vi "VISJS Viewer.vi"(4 "Extra Scripts":string, 5 "FileDependency In":map{path, T1}(c390), 6 "Options":string, 7 "OpenWebBrowser(False)":bool, 8 "error in":errorcluster, 9 "Embedd VISJS Librarya in HTMl File(False)":bool, 10 "HTMLFilePath":path, 11 "LibraryDependency":map{path, T3}(c390)) -> (0 "error out":errorcluster, 3 "HTMLFileContent":string)   [LabVIEW 2020, in "VISJS Viewer.lvlib"] (continued)
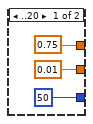
[diagram p2: hidden frame]
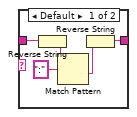
[diagram p7: hidden frame]
d=r[2];e<s&&(e=s,C=n,I=a,i=d)}}return[C,e,I,i]}},{key:\"_getEnergy\",value:function(g){var t=lh(this.E_sums[g],2),A=t[0],e=t[1];return[Math.sqrt(Math.pow(A,2)+Math.pow(e,2)),A,e]}},{key:\"_moveNode\",value:function(g,t,A){for(var e=this.body.nodeIndices,C=this.body.nodes,I=0,i=0,o=0,n=C[g].x,r=C[g].y,s=this.K_matrix[g],a=this.L_matrix[g],d=0;d<e.length;d++){var h=e[d];if(h!==g){var l=C[h].x,c=C[h].y,u=s[h],p=a[h],f=1/Math.pow(Math.pow(n-l,2)+Math.pow(r-c,2),1.5);I+=u*(1-p*Math.pow(r-c,2)*f),i+=u*(p*(n-l)*(r-c)*f),o+=u*(1-p*Math.pow(n-l,2)*f)}}var v=(t/I+A/i)/(i/I-o/i),y=-(i*v+t)/I;C[g].x+=y,C[g].y+=v,this._updateE_matrix(g)}},{key:\"_createL_matrix\",value:function(g){var t=this.body.nodeIndices,A=this.springLength;this.L_matrix=[];for(var e=0;e<t.length;e++){this.L_matrix[t[e]]={};for(var C=0;C<t.length;C++)this.L_matrix[t[e]][t[C]]=A*g[t[e]][t[C]]}}},{key:\"_createK_matrix\",value:function(g){var t=this.body.nodeIndices,A=this.springConstant;this.K_matrix=[];for(var e=0;e<t.length;e++){this.K_matrix[t[e]]={};for(var C=0;C<t.length;C++)this.K_matrix[t[e]][t[C]]=A*Math.pow(g[t[e]][t[C]],-2)}}},{key:\"_createE_matrix\",value:function(){var g=this.body.nodeIndices,t=this.body.nodes;this.E_matrix={},this.E_sums={};for(var A=0;A<g.length;A++)this.E_matrix[g[A]]=[];for(var e=0;e<g.length;e++){for(var C=g[e],I=t[C].x,i=t[C].y,o=0,n=0,r=e;r<g.length;r++){var s=g[r];if(s!==C){var a=t[s].x,d=t[s].y,h=1/Math.sqrt(Math.pow(I-a,2)+Math.pow(i-d,2));this.E_matrix[C][r]=[this.K_matrix[C][s]*(I-a-this.L_matrix[C][s]*(I-a)*h),this.K_matrix[C][s]*(i-d-this.L_matrix[C][s]*(i-d)*h)],this.E_matrix[s][e]=this.E_matrix[C][r],o+=this.E_matrix[C][r][0],n+=this.E_matrix[C][r][1]}}this.E_sums[C]=[o,n]}}},{key:\"_updateE_matrix\",value:function(g){for(var t=this.body.nodeIndices,A=this.body.nodes,e=this.E_matrix[g],C=this.K_matrix[g],I=this.L_matrix[g],i=A[g].x,o=A[g].y,n=0,r=0,s=0;s<t.length;s++){var a=t[s];if(a!==g){var d=e[s],h=d[0],l=d[1],c=A[a].x,u=A[a].y,p=1/Math.sqrt(Math.pow(i-c,2)+Math.pow(o-u,2)),f=C[a]*(i-c-I[a]*(i-c)*p),v=C[a]*(o-u-I[a]*(o-u)*p);e[s]=[f,v],n+=f,r+=v;var y=this.E_sums[a];y[0]+=f-h,y[1]+=v-l}}this.E_sums[g]=[n,r]}}]),g}();function gB(g,t,A){var e,C,I,i,o=this;if(!(this instanceof gB))throw new SyntaxError(\"Constructor must be called with the new operator\");this.options={},this.defaultOptions={locale:\"en\",locales:ny,clickToUse:!1},fe(this.options,this.defaultOptions),this.body={container:g,nodes:{},nodeIndices:[],edges:{},edgeIndices:[],emitter:{on:je(e=this.on).call(e,this),off:je(C=this.off).call(C,this),emit:je(I=this.emit).call(I,this),once:je(i=this.once).call(i,this)},eventListeners:{onTap:function(){},onTouch:function(){},onDoubleTap:function(){},onHold:function(){},onDragStart:function(){},onDrag:function(){},onDragEnd:function(){},onMouseWheel:function(){},onPinch:function(){},onMouseMove:function(){},onRelease:function(){},onContext:function(){}},data:{nodes:null,edges:null},functions:{createNode:function(){},createEdge:function(){},getPointer:function(){}},modules:{},view:{scale:1,translation:{x:0,y:0}},selectionBox:{show:!1,position:{start:{x:0,y:0},end:{x:0,y:0}}}},this.bindEventListeners(),this.images=new sy((function(){return o.body.emitter.emit(\"_requestRedraw\")})),this.groups=new Gm,this.canvas=new CP(this.body),this.selectionHandler=new yM(this.body,this.canvas),this.interactionHandler=new sP(this.body,this.canvas,this.selectionHandler),this.view=new IP(this.body,this.canvas),this.renderer=new gP(this.body,this.canvas),this.physics=new HR(this.body),this.layoutEngine=new ZM(this.body),this.clustering=new $R(this.body),this.manipulation=new jM(this.body,this.canvas,this.selectionHandler,this.interactionHandler),this.nodesHandler=new YN(this.body,this.images,this.groups,this.layoutEngine),this.edgesHandler=new FR(this.body,this.images,this.groups),this.body.modules.kamadaKawai=new $M(this.body,150,.05),this.body.modules.clustering=this.clustering,this.canvas._create(),this.setOptions(A),this.setData(t)}He(gB.prototype),gB.prototype.setOptions=function(g){var t=this;if(null===g&&(g=void 0),void 0!==g){!0===Dv.validate(g,KM)&&console.error(\"%cErrors have been found in the supplied options object.\",Tv);if(Xf([\"locale\",\"locales\",\"clickToUse\"],this.options,g),void 0!==g.locale&&(g.locale=function(g,t){try{var A=lh(t.split(/[-_ /]/,2),2),e=A[0],C=A[1],I=null!=e?e.toLowerCase():null,i=null!=C?C.toUpperCase():null;if(I&&i){var o,n=I+\"-\"+i;if(Object.prototype.hasOwnProperty.call(g,n))return n;console.warn(bh(o=\"Unknown variant \".concat(i,\" of language \")).call(o,I,\".\"))}if(I){var r=I;if(Object.prototype.hasOwnProperty.call(g,r))return r;console.warn(\"Unknown language \".concat(I))}return console.warn(\"Unknown locale \".concat(t,\", falling back to English.\")),\"en\"}catch(g){return console.error(g),console.warn(\"Unexpected error while normalizing locale \".concat(t,\", falling back to English.\")),\"en\"}}(g.locales||this.options.locales,g.locale)),g=this.layoutEngine.setOptions(g.layout,g),this.canvas.setOptions(g),this.groups.setOptions(g.groups),this.nodesHandler.setOptions(g.nodes),this.edgesHandler.setOptions(g.edges),this.physics.setOptions(g.physics),this.manipulation.setOptions(g.manipulation,g,this.options),this.interactionHandler.setOptions(g.interaction),this.renderer.setOptions(g.interaction),this.selectionHandler.setOptions(g.interaction),void 0!==g.groups&&this.body.emitter.emit(\"refreshNodes\"),\"configure\"in g&&(this.configurator||(this.configurator=new xv(this,this.body.container,HM,this.canvas.pixelRatio,XM)),this.configurator.setOptions(g.configure)),this.configurator&&!0===this.configurator.options.enabled){var A={nodes:{},edges:{},layout:{},interaction:{},manipulation:{},physics:{},global:{}};qf(A.nodes,this.nodesHandler.options),qf(A.edges,this.edgesHandler.options),qf(A.layout,this.layoutEngine.options),qf(A.interaction,this.selectionHandler.options),qf(A.interaction,this.renderer.options),qf(A.interaction,this.interactionHandler.options),qf(A.manipulation,this.manipulation.options),qf(A.physics,this.physics.options),qf(A.global,this.canvas.options),qf(A.global,this.options),this.configurator.setModuleOptions(A)}void 0!==g.clickToUse?!0===g.clickToUse?void 0===this.activator&&(this.activator=new kv(this.canvas.frame),this.activator.on(\"change\",(function(){t.body.emitter.emit(\"activate\")}))):(void 0!==this.activator&&(this.activator.destroy(),delete this.activator),this.body.emitter.emit(\"activate\")):this.body.emitter.emit(\"activate\"),this.canvas.setSize(),this.body.emitter.emit(\"startSimulation\")}},gB.prototype._updateVisibleIndices=function(){var g=this.body.nodes,t=this.body.edges;for(var A in this.body.nodeIndices=[],this.body.edgeIndices=[],g)Object.prototype.hasOwnProperty.call(g,A)&&(this.clustering._isClusteredNode(A)||!1!==g[A].options.hidden||this.body.nodeIndices.push(g[A].id));for(var e in t)if(Object.prototype.hasOwnProperty.call(t,e)){var C=t[e],I=g[C.fromId],i=g[C.toId],o=void 0!==I&&void 0!==i;!this.clustering._isClusteredEdge(e)&&!1===C.options.hidden&&o&&!1===I.options.hidden&&!1===i.options.hidden&&this.body.edgeIndices.push(C.id)}},gB.prototype.bindEventListeners=function(){var g=this;this.body.emitter.on(\"_dataChanged\",(function(){g.edgesHandler._updateState(),g.body.emitter.emit(\"_dataUpdated\")})),this.body.emitter.on(\"_dataUpdated\",(function(){g.clustering._updateState(),g._updateVisibleIndices(),g._updateValueRange(g.body.nodes),g._updateValueRange(g.body.edges),g.body.emitter.emit(\"startSimulation\"),g.body.emitter.emit(\"_requestRedraw\")}))},gB.prototype.setData=function(g){if(this.body.emitter.emit(\"resetPhysics\"),this.body.emitter.emit(\"_resetData\"),this.selectionHandler.unselectAll(),g&&g.dot&&(g.nodes||g.edges))throw new SyntaxError('Data must contain either parameter \"dot\" or  parameter pair \"nodes\" and \"edges\", but not both.');if(this.setOptions(g&&g.options),g&&g.dot){console.warn(\"The dot property has been deprecated. Please use the static convertDot method to convert DOT into vis.network format and use the normal data format with nodes and edges. This converter is used like this: var data = vis.network.convertDot(dotString);\");var t=Cy(g.dot);this.setData(t)}else if(g&&g.gephi){console.warn(\"The gephi property has been deprecated. Please use the static convertGephi method to convert gephi into vis.network format and use the normal data format with nodes and edges. This converter is used like this: var data = vis.network.convertGephi(gephiJson);\");var A=iy(g.gephi);this.setData(A)}else this.nodesHandler.setData(g&&g.nodes,!0),this.edgesHandler.setData(g&&g.edges,!0),this.body.emitter.emit(\"_dataChanged\"),this.body.emitter.emit(\"_dataLoaded\"),this.body.emitter.emit(\"initPhysics\")},gB.prototype.destroy=function(){for(var g in this.body.emitter.emit(\"destroy\"),this.body.emitter.off(),this.off(),delete this.groups,delete this.canvas,delete this.selectionHandler,delete this.interactionHandler,delete this.view,delete this.renderer,delete this.physics,delete this.layoutEngine,delete this.clustering,delete this.manipulation,delete this.nodesHandler,delete this.edgesHandler,delete this.configurator,delete this.images,this.body.nodes)Object.prototype.hasOwnProperty.call(this.body.nodes,g)&&delete this.body.nodes[g];for(var t in this.body.edges)Object.prototype.hasOwnProperty.call(this.body.edges,t)&&delete this.body.edges[t];Qf(this.body.container)},gB.prototype._updateValueRange=function(g){var t,A=void 0,e=void 0,C=0;for(t in g)if(Object.prototype.hasOwnProperty.call(g,t)){var I=g[t].getValue();void 0!==I&&(A=void 0===A?I:Math.min(I,A),e=void 0===e?I:Math.max(I,e),C+=I)}if(void 0!==A&&void 0!==e)for(t in g)Object.prototype.hasOwnProperty.call(g,t)&&g[t].setValueRange(A,e,C)},gB.prototype.isActive=function(){return!this.activator||this.activator.active},gB.prototype.setSize=function(){return this.canvas.setSize.apply(this.canvas,arguments)},gB.prototype.canvasToDOM=function(){return this.canvas.canvasToDOM.apply(this.canvas,arguments)},gB.prototype.DOMtoCanvas=function(){return this.canvas.DOMtoCanvas.apply(this.canvas,arguments)},gB.prototype.findNode=function(){return this.clustering.findNode.apply(this.clustering,arguments)},gB.prototype.isCluster=function(){return this.clustering.isCluster.apply(this.clustering,arguments)},gB.prototype.openCluster=function(){return this.clustering.openCluster.apply(this.clustering,arguments)},gB.prototype.cluster=function(){return this.clustering.cluster.apply(this.clustering,arguments)},gB.prototype.getNodesInCluster=function(){return this.clustering.getNodesInCluster.apply(this.clustering,arguments)},gB.prototype.clusterByConnection=function(){return this.clustering.clusterByConnection.apply(this.clustering,arguments)},gB.prototype.clusterByHubsize=function(){return this.clustering.clusterByHubsize.apply(this.clustering,arguments)},gB.prototype.updateClusteredNode=function(){return this.clustering.updateClusteredNode.apply(this.clustering,arguments)},gB.prototype.getClusteredEdges=function(){return this.clustering.getClusteredEdges.apply(this.clustering,arguments)},gB.prototype.getBaseEdge=function(){return this.clustering.getBaseEdge.apply(this.clustering,arguments)},gB.prototype.getBaseEdges=function(){return this.clustering.getBaseEdges.apply(this.clustering,arguments)},gB.prototype.updateEdge=function(){return this.clustering.updateEdge.apply(this.clustering,arguments)},gB.prototype.clusterOutliers=function(){return this.clustering.clusterOutliers.apply(this.clustering,arguments)},gB.prototype.getSeed=function(){return this.layoutEngine.getSeed.apply(this.layoutEngine,arguments)},gB.prototype.enableEditMode=function(){return this.manipulation.enableEditMode.apply(this.manipulation,arguments)},gB.prototype.disableEditMode=function(){return this.manipulation.disableEditMode.apply(this.manipulation,arguments)},gB.prototype.addNodeMode=function(){return this.manipulation.addNodeMode.apply(this.manipulation,arguments)},gB.prototype.editNode=function(){return this.manipulation.editNode.apply(this.manipulation,arguments)},gB.prototype.editNodeMode=function(){return console.warn(\"Deprecated: Please use editNode instead of editNodeMode.\"),this.manipulation.editNode.apply(this.manipulation,arguments)},gB.prototype.addEdgeMode=function(){return this.manipulation.addEdgeMode.apply(this.manipulation,arguments)},gB.prototype.editEdgeMode=function(){return this.manipulation.editEdgeMode.apply(this.manipulation,arguments)},gB.prototype.deleteSelected=function(){return this.manipulation.deleteSelected.apply(this.manipulation,arguments)},gB.prototype.getPositions=function(){return this.nodesHandler.getPositions.apply(this.nodesHandler,arguments)},gB.prototype.getPosition=function(){return this.nodesHandler.getPosition.apply(this.nodesHandler,arguments)},gB.prototype.storePositions=function(){return this.nodesHandler.storePositions.apply(this.nodesHandler,arguments)},gB.prototype.moveNode=function(){return this.nodesHandler.moveNode.apply(this.nodesHandler,arguments)},gB.prototype.getBoundingBox=function(){return this.nodesHandler.getBoundingBox.apply(this.nodesHandler,arguments)},gB.prototype.getConnectedNodes=function(g){return void 0!==this.body.nodes[g]?this.nodesHandler.getConnectedNodes.apply(this.nodesHandler,arguments):this.edgesHandler.getConnectedNodes.apply(this.edgesHandler,arguments)},gB.prototype.getConnectedEdges=function(){return this.nodesHandler.getConnectedEdges.apply(this.nodesHandler,arguments)},gB.prototype.startSimulation=function(){return this.physics.startSimulation.apply(this.physics,arguments)},gB.prototype.stopSimulation=function(){return this.physics.stopSimulation.apply(this.physics,arguments)},gB.prototype.stabilize=function(){return this.physics.stabilize.apply(this.physics,arguments)},gB.prototype.getSelection=function(){return this.selectionHandler.getSelection.apply(this.selectionHandler,arguments)},gB.prototype.setSelection=function(){return this.selectionHandler.setSelection.apply(this.selectionHandler,arguments)},gB.prototype.getSelectedNodes=function(){return this.selectionHandler.getSelectedNodeIds.apply(this.selectionHandler,arguments)},gB.prototype.getSelectedEdges=function(){return this.selectionHandler.getSelectedEdgeIds.apply(this.selectionHandler,arguments)},gB.prototype.getNodeAt=function(){var g=this.selectionHandler.getNodeAt.apply(this.selectionHandler,arguments);return void 0!==g&&void 0!==g.id?g.id:g},gB.prototype.getEdgeAt=function(){var g=this.selectionHandler.getEdgeAt.apply(this.selectionHandler,arguments);return void 0!==g&&void 0!==g.id?g.id:g},gB.prototype.selectNodes=function(){return this.selectionHandler.selectNodes.apply(this.selectionHandler,arguments)},gB.prototype.selectEdges=function(){return this.selectionHandler.selectEdges.apply(this.selectionHandler,arguments)},gB.prototype.unselectAll=function(){this.selectionHandler.unselectAll.apply(this.selectionHandler,arguments),this.selectionHandler.commitWithoutEmitting.apply(this.selectionHandler),this.redraw()},gB.prototype.redraw=function(){return this.renderer.redraw.apply(this.renderer,arguments)},gB.prototype.getScale=function(){return this.view.getScale.apply(this.view,arguments)},gB.prototype.getViewPosition=function(){return this.view.getViewPosition.apply(this.view,arguments)},gB.prototype.fit=function(){return this.view.fit.apply(this.view,arguments)},gB.prototype.moveTo=function(){return this.view.moveTo.apply(this.view,arguments)},gB.prototype.focus=function(){return this.view.focus.apply(this.view,arguments)},gB.prototype.releaseNode=function(){return this.view.releaseNode.apply(this.view,arguments)},gB.prototype.getOptionsFromConfigurator=function(){var g={};return this.configurator&&(g=this.configurator.getOptions.apply(this.configurator)),g};var tB=Cy;g.DataSet=mD,g.DataView=bD,g.Network=gB,g.NetworkImages=sy,g.Queue=fD,g.data=xD,g.networkDOTParser=Iy,g.networkGephiParser=oy,g.networkOptions=JM,g.parseDOTNetwork=tB,g.parseGephiNetwork=iy}));\n//# sourceMappingURL=vis-network.min.js.map\n"  # https://visjs.github.io/vis-network/standalone/umd/vis-network.min.js 2024-08-26T06:20:20.413Z
  n1 = Array Size(array=w28) -> (size(s)=w29:i32)
  n2 = for {
    tunnel: "LibraryDependency" -> [w51] mode=indexing
    tunnel: "{from: \"%s\",to: \"%s\",arrows: \"to\",id: \"E%d\"}\n" -> [w49]
    tunnel: [w44] -> w25 mode=concatenating
    shift-right: [w42] -> _
    shift-left: 0 -> [w48]
    tunnel: "FileDependency In" -> [w47]
    tunnel: [w43] -> w4 mode=concatenating
    tunnel: [w46] -> _ mode=indexing
    i -> [w46]
    n3 = Unbundle By Name(w51) -> ("LibraryDependentInfo.ParentLibraries"=w41:path[], "Path"=w45:path, "LibraryDependentInfo.DependentLibrary"=w50:map{path, set{path}})  [unwired: 1 out]
    n4 = for {
      tunnel: w45 -> [w72]
      tunnel: w50 -> [w69] mode=indexing
      tunnel: w49 -> [w71]
      tunnel: [w70] -> w44 mode=indexing
      shift-right: [w55] -> w42
      shift-left: w48 -> [w66]
      tunnel: w47 -> [w65]
      tunnel: [w62] -> w43 mode=indexing
      tunnel: w41 -> [w57]
      n5 = Unbundle By Name(w69) -> ("Path"=w56:path, "Callers"=w64:set{path})
      n6 = for {
        tunnel: w65 -> [w98]
        tunnel: w64 -> [w97] mode=indexing
        shift-right: [w93] -> w60
        shift-left: map{string, set{string}} {} ("Size: 0") -> [w95]
        n7 = Look In Map(map=w98, key=w97) -> (value=w96:T1)  [unwired: 1 in, 1 out]
        n8 = Unbundle By Name(w96) -> ("FullQualifierName"=w90:string, "Path"=w92:path)
        n9 = call <vilib>:"Get File Extension.vi"("file"=w92) -> ("lowercase file extension"=w91:string)  [unwired: 6 in, 4 out]
        n10 = case shown="\"lvclass\"" w91 {
          tunnel: w90 -> [w103 w104]
          tunnel: [w99 w104] -> w89
          frame Default {
            n11 = Reverse String(1:w103) -> (0:w102:string)
            n12 = Match Pattern(string=w102, regular expression=":") -> (after substring=w100:string)  [unwired: 1 in, 3 out]
            n13 = Reverse String(1:w100) -> (0:w99:string)
          }
          frame "lvclass" {
          }
        }
        n14 = Strip Path(path=w92) -> (name=w94:string)  [unwired: 1 out]
        n15 = in-place {
          in-place-border: w94 -> [w107]
          n16 = in-place-map #1(w95, w89) -> (w108:set{string})  [unwired: 1 in, 1 out]
          n17 = Insert Into Set(10:w107, 11:w108) -> (3:w106:set{string})  [unwired: 1 out]
          n18 = in-place-map #1(w106, LVMapReplaceAction."Add or Modify Entry" ("action")) -> (w93:map{string, set{string}})  [unwired: 2 out]
        }
      }
      n19 = Search 1D Array(1D array=w57, element=w56) -> (index of element=w53:i32)  [unwired: 1 in]
      n20 = case shown="0, Default" w53 {
        tunnel: ["INHERITANCE " _] -> w52
        frame 0, Default {
        }
        frame -1 {
        }
      }
      n21 = Increment(x=w66) -> (x+1=w55:i32)
      n22 = for {
        tunnel: w60 -> [w80] mode=indexing
        tunnel: [w77] -> w59 mode=indexing
        n23 = Unbundle(w80) -> ("FullQualifierName"=w75:string, w79:set{string})
        n24 = for {
          tunnel: w79 -> [w88] mode=indexing
          tunnel: [w88] -> w78 mode=indexing if=w86
          tunnel: w75 -> [w87]
          n25 = Not Equal?(x=w87, y=w88) -> (x != y?=w86:bool)
        }
        n26 = call <vilib>:"Join Strings.vi"("Separator (,)"=", ", "Strings In"=w78) -> ("String"=w76:string)  [unwired: 1 in]
        n27 = case shown="Default" w75 {
          selector: w75 -> [_ w85]
          tunnel: w76 -> [w81 w83]
          tunnel: [w81 w82] -> w77
          frame "" {
          }
          frame Default {
            n28 = Format Into String(format string="%s  [%s]", w85, w83) -> (resulting string=w82:string)  [unwired: 2 in, 1 out]
          }
        }
      }
      n29 = call "VISJS Viewer_EscapePath.vi"("Path"=w72) -> ("File Path"=w68:string)  [unwired: 10 in]
      n30 = call "VISJS Viewer_EscapePath.vi"("Path"=w56) -> ("File Path"=w67:string)  [unwired: 10 in]
      n31 = call <vilib>:"Join Strings.vi"("Separator (,)"="<BR> ", "Strings In"=w59) -> ("String"=w54:string)  [unwired: 1 in]
      n32 = Format Into String(format string="E%d : \"%s%s\"\n", w55, w52, w54) -> (resulting string=w62:string)  [unwired: 2 in, 1 out]
      n33 = Format Into String(format string=w71, w68, w67, w55) -> (resulting string=w70:string)  [unwired: 2 in, 1 out]
    }
  }
  n34 = for {
    tunnel: "LibraryDependency" -> [w127] mode=indexing
    tunnel: "{id: \"%s\",size: 150,label:\"%s\",color: \"#%02X%02X%02x\",cid: \"%s\",shape: \"box\"}\n" -> [w126]
    tunnel: w29 -> [w124]
    tunnel: w28 -> [w122]
    tunnel: [w116] -> w27 mode=indexing
    i -> [w125]
    w110 = ":" ("search string")
    n35 = Unbundle By Name(w127) -> ("Path"=w121:path, "LibraryDependentInfo.FullQualifierName"=w111:string)
    n36 = Quotient & Remainder(x=w125, y=w124) -> (x-y*floor(x/y)=w123:i32)  [unwired: 1 out]
    n37 = Index Array(array=w122, index=w123) -> (element=w120:u32)
    n38 = call <vilib>:"Color to RGB.vi"("Color"=w120) -> ("R"=w119:u8, "G"=w118:u8, "B"=w117:u8)  [unwired: 1 out]
    n39 = Match Pattern(string=w111, regular expression=w110) -> (before substring=w109:string)  [unwired: 1 in, 3 out]
    n40 = Search and Replace String(replace all?=TRUE ("replace all? (F)"), input string=w111, search string=w110, replace string="\\n" ("replace string (\"\")")) -> (result string=w113:string)  [unwired: 4 in, 3 out]
    n41 = call "VISJS Viewer_EscapePath.vi"("Path"=w121) -> ("File Path"=w115:string)  [unwired: 10 in]
    n42 = Format Into String(format string=w126, w115, w113, w119, w118, w117, w109) -> (resulting string=w116:string)  [unwired: 2 in, 1 out]
  }
  n43 = Empty String/Path?(string/path="HTMLFilePath") -> (empty?=w36:bool)
  n44 = Compound Arithmetic op=AND(w36, "OpenWebBrowser(False)") -> (w35:bool)
  n45 = Collection Size(1:"LibraryDependency") -> (0:w11:i32)
  n46 = case shown="21.." w11 {
    tunnel: [0.75 0.75] -> w8
    tunnel: [0.01 0.01] -> w7
    tunnel: [50 125] -> w6
    frame ..20 {
    }
    frame 21.. {
    }
  }
  n47 = case shown="True" w35 {
    tunnel: "HTMLFilePath" -> [w134 _]
    tunnel: [w134 w135] -> w18
    frame False {
    }
    frame True {
      n48 = Temporary Directory() -> (w137:path)
      n49 = Build Path(base path=w137, name or relative path=path "VISJS_Viewer.html") -> (appended path=w135:path)
    }
  }
  n50 = Format Into String(format string=w9, w8, w7, w6) -> (resulting string=w10:string)  [unwired: 2 in, 1 out]
  n51 = call <vilib>:"Join Strings.vi"("Strings In"=w27) -> ("String"=w26:string)  [unwired: 2 in]
  n52 = Select(t=w39, s="Embedd VISJS Librarya in HTMl File(False)", f="<script src=\"https://visjs.github.io/vis-network/standalone/umd/vis-network.min.js\"></script>") -> (s? t:f=w32:string)
  n53 = Empty String/Path?(string/path="Options") -> (empty?=w15:bool)
  n54 = Select(t=w10, s=w15, f="Options") -> (s? t:f=w13:string)
  n55 = call <vilib>:"Join Strings.vi"("Strings In"=w25) -> ("String"=w24:string)  [unwired: 2 in]
  n56 = call <vilib>:"Join Strings.vi"("Strings In"=w4) -> ("String"=w3:string)  [unwired: 2 in]
  n57 = Build Array(w32, w13, w26, w24, "Extra Scripts", w3) -> (w31:string[])
  n58 = for {
    shift-right: [w140] -> w17
    shift-left: "\n<html lang=\"en\">\n  <head>\n    <title>Vis Network | Example Applications | Disassembler</title>\n    <style type=\"text/css\">\n      #mynetwork {\n        width: 100%;\n        height: 80vh; /* Adjust height so the information appears at the bottom */\n        border: 0px solid lightgray;\n      }\n      #edgeInfo {\n        padding: 10px;\n        background-color: #f9f9f9;\n        border-top: 1px solid #ddd;\n      }\n\n /* Context menu styles */\n    .context-menu {\n      position: absolute;\n      display: none;\n      background-color: white;\n      border: 1px solid #ccc;\n      z-index: 100;\n      padding: 10px;\n      box-shadow: 2px 2px 5px rgba(0,0,0,0.2);\n    }\n\n    .context-menu button {\n      display: block;\n      background: none;\n      border: none;\n      padding: 5px 10px;\n      text-align: left;\n      width: 100%;\n      cursor: pointer;\n    }\n\n    .context-menu button:hover {\n      background-color: #f1f1f1;\n    }\n\n    #selectionBox {\n      position: absolute;\n      border: 1px dashed #555;\n      background: rgba(0, 0, 255, 0.1);\n      display: none;\n    }\n    </style>\n    <<VISJS>>\n  </head>\n  <body>\n    <div id=\"mynetwork\"></div>\n    <div id=\"selectionBox\"></div>\n    <div id=\"contextMenu\" class=\"context-menu\">\n      <button id=\"togglePhysics\">Toggle Physics</button>\n    </div>\n    <div id=\"edgeInfo\">Click on a node or edge to view its dependency details.<BR>Right-click on a node to turn the physics on or off for that node.<BR>To select multiple nodes, hold Shift and drag with a left click.</div>\n    <script type=\"text/javascript\">\n\nconst options = {\n<<OPTIONS>>\n};\n\nvar nodes = new vis.DataSet([\n<<NODES>>\n]);\n\n\nvar edges = new vis.DataSet([\n<<EDGES>>\n]);\n\nconst edgeInfoMap = {\n <<EDGEDEPENDECY>>\n};\n\n\n      var container = document.getElementById(\"mynetwork\");\n      var data = { nodes: nodes, edges: edges };\n      var gph = new vis.Network(container, data, options);\n      var contextMenu = document.getElementById('contextMenu');\n      var selectedNodeId = null;\n      var selectionBox = document.getElementById('selectionBox');\n      var startX, startY, isSelecting = false;\n\n      // Show context menu on right-click\n      gph.on(\"oncontext\", function (params) {\n        params.event.preventDefault();\n        var nodeId = gph.getNodeAt(params.pointer.DOM);\n\n        if (nodeId !== undefined) {\n          selectedNodeId = nodeId;\n          contextMenu.style.left = params.event.pageX + \"px\";\n          contextMenu.style.top = params.event.pageY + \"px\";\n          contextMenu.style.display = \"block\";\n        }\n      });\n\n      // Hide context menu when clicking anywhere\n      document.addEventListener(\"click\", function () {\n        contextMenu.style.display = \"none\";\n      });\n\n    document.getElementById('togglePhysics').addEventListener('click', function () {\n        if (selectedNodeId !== null) {\n        var node = nodes.get(selectedNodeId);\n        \n        // Toggle the physics state\n        if (node.physics === undefined || node.physics === null) node.physics = true;\n        node.physics = !node.physics;\n\n        // Update the node with the new fixed state\n                nodes.update(node);\n\n        selectedNodeId = null;\n        contextMenu.style.display = \"none\";\n        }\n    });\n\n    // Capture mousedown to start selection\n    container.addEventListener('mousedown', function(event) {\n    startX = event.clientX;\n    startY = event.clientY;\n    selectionBox.style.left = startX + 'px';\n    selectionBox.style.top = startY + 'px';\n    selectionBox.style.width = '0px';\n    selectionBox.style.height = '0px';\n    selectionBox.style.display = 'block';\n    isSelecting = true;\n  });\n\n  // Capture mousemove to draw the selection box\n  container.addEventListener('mousemove', function(event) {\n    if (isSelecting) {\n      var currentX = event.clientX;\n      var currentY = event.clientY;\n      selectionBox.style.left = Math.min(startX, currentX) + 'px';\n      selectionBox.style.top = Math.min(startY, currentY) + 'px';\n      selectionBox.style.width = Math.abs(currentX - startX) + 'px';\n      selectionBox.style.height = Math.abs(currentY - startY) + 'px';\n    }\n  });\n\n  // Capture mouseup to end selection and select nodes\n  container.addEventListener('mouseup', function(event) {\n    if (isSelecting) {\n      var endX = event.clientX;\n      var endY = event.clientY;\n\n      var selectionRect = {\n        left: Math.min(startX, endX),\n        right: Math.max(startX, endX),\n        top: Math.min(startY, endY),\n        bottom: Math.max(startY, endY)\n      };\n\n      var selectedNodes = [];\n      nodes.forEach(function(node) {\n        var nodePosition = gph.getPositions([node.id])[node.id];\n        var canvasPosition = gph.canvasToDOM(nodePosition);\n\n        // Check if node is inside the selection box\n        if (canvasPosition.x >= selectionRect.left && canvasPosition.x <= selectionRect.right &&\n            canvasPosition.y >= selectionRect.top && canvasPosition.y <= selectionRect.bottom) {\n          selectedNodes.push(node.id);\n        }\n      });\n\n      // Highlight selected nodes\n      gph.selectNodes(selectedNodes);\n      selectionBox.style.display = 'none';\n      isSelecting = false;\n    }\n  });\n\n  // Optional: Reset selection box on mouse leave\n  container.addEventListener('mouseleave', function() {\n    selectionBox.style.display = 'none';\n    isSelecting = false;\n  });\n/*\ngph.fit({\n animation: false, // Smooth transition\n minZoomLevel: .1, // Prevent zooming out too far\n maxZoomLevel: 10  // Allow zooming in more\n});\n*/\n   gph.on(\"click\", function (params) {\n  const edgeInfoElement = document.getElementById(\"edgeInfo\");\n  \n  // Check if a node is clicked\n  const nodeId = this.getNodeAt(params.pointer.DOM);\n  if (nodeId) {\n    // Get all edges where the nodeId is the \"from\" node\n    const connectedEdges = edges.get({\n      filter: (edge) => edge.from === nodeId,\n    });\n\nif (connectedEdges.length > 0) {\n  let allEdgeInfo = \"\";\n  connectedEdges.forEach((edge, index) => {\n    const edgeInfo = edgeInfoMap[edge.id] || \"No info available for this edge.\";\n    const bgColor = index % 2 === 0 ? \"#f0f0f0\" : \"#ffffff\"; // Alternate background color\n    allEdgeInfo += `<div style=\"background-color: ${bgColor}; padding: 5px;\">${edgeInfo}</div>`;\n  });\n  edgeInfoElement.innerHTML = allEdgeInfo;\n} else {\n      edgeInfoElement.innerHTML = \"No outgoing edges from this node.\";\n    }\n    return;\n  }\n\n  // Check if an edge is clicked\n  const edgeId = this.getEdgeAt(params.pointer.DOM);\n  if (edgeId) {\n    edgeInfoElement.innerHTML = edgeInfoMap[edgeId] || \"No info available for this edge.\";\n    return;\n  }\n\n  // Default message if neither node nor edge is clicked\n  edgeInfoElement.innerHTML = \"Click on a node or edge to view its dependency details.<BR>Right-click on a node to turn the physics on or off for that node.<BR>To select multiple nodes, hold Shift and drag with a left click.\";\n});\n\n\n<<EXTRASCRIPTS>>\n    </script>\n  </body>\n</html>\n" -> [w141]
    tunnel: string[] [" <<VISJS>>", "<<OPTIONS>>", "<<NODES>>", "<<EDGES>>", "<<EXTRASCRIPTS>>", " <<EDGEDEPENDECY>>"] -> [w139] mode=indexing
    tunnel: w31 -> [w138] mode=indexing
    n59 = Search and Replace String(input string=w141, search string=w139, replace string=w138) -> (result string=w140:string)  [unwired: 5 in, 3 out]
  }
  "HTMLFileContent" <- w17
  n60 = Empty String/Path?(string/path=w18) -> (empty?=w23:bool)
  n61 = case shown="False" w23 {
    tunnel: w18 -> [w145 _]
    tunnel: "error in" -> [w144 w146]
    tunnel: [w143 w146] -> w21
    tunnel: w17 -> [w142 _]
    frame False {
      n62 = Write to Text File(file (use dialog)=w145, text=w142, error in=w144) -> (error out=w143:errorcluster)  [unwired: 1 in, 2 out]
    }
    frame True {
    }
  }
  n63 = case shown="True" "OpenWebBrowser(False)" {
    tunnel: w21 -> [w147 w150]
    tunnel: [w147 w149] -> w20
    tunnel: w18 -> [_ w148]
    frame False {
    }
    frame True {
      n64 = call-poly <vilib>:"Open URL in Default Browser.vi"("error in (no error)"=w150, "path"=w148) -> ("error out"=w149:errorcluster)  [unwired: 4 in, 1 out]
    }
  }
  "error out" <- w20
